vi "AVS_Main.vi"() -> ()   [LabVIEW 2009]
uses:
  <vilib>/express/express arith-compare/Formula/XNode/ExpressFormulaBlockNode.xnode
  Instance           4 16Saved   AVS_Main .vi
  Instance           6 16Saved   AVS_Main .vi
  Instance           5 16Saved   AVS_Main .vi
panel:
  out "a_hDevice":i32
  out "StartTime":u32
  out "XY Graph":cluster{"Y":dbl[], "Y":dbl[]}[](graph)
  out "LastScanTime":dbl caption="Last scan in [ms]" format="%#4.2f"
  out "AvgTimePerScan":dbl caption="Avg Time /Scan [ms]" format="%#4.2f"
  out "Failures":dbl caption="Nr Of Failures" format="%#.0f"
  out "PerformedScans":dbl caption="Nr Of Scans" format="%#.0f"
  out "TotalTime":dbl caption="Time Since Start [s]" format="%#.1f"
  in  "StopMeasurement":bool
  out "Status":string
  in  "StartMeasurement":bool caption="Start Measurement"
  in  "NrOfScans":i16 caption="Nr Of Scans"
  in  "RamSpectra":u16 caption="Spectra stored to RAM"
  in  "LaserWavelenght":sgl caption="Laser Wavelenght [nm]" format="%.2f"
  in  "LaserWidth":u32 caption="Laser Width [ns]"
  in  "LaserDelay":u32 caption="Laser Delay [ns]"
  in  "FlashesPerScan":u16 caption="Flashes per Scan"
  in  "SmoothModel":u8 caption="Model"
  in  "SmoothPix":u16 caption="Nr Of Pixels"
  in  "EnableDarkCorrection":bool caption="Enable"
  in  "DarkHist":u8 caption="%"
  in  "SatDetection":u8 caption="Saturation detection"
  in  "NrOfAVG":u32 caption="Number of averages"
  in  "IntDelay":dbl caption="Integration delay [ns]" min=-20.0 format="%#.0f"
  in  "IntTime":sgl caption="Integration time [ms]" format="%.2f"
  in  "StartPixel":u16 caption="Start pixel"
  in  "StopPixel":u16 caption="Stop pixel"
  in  "Trigger type":enum32{"Radio Selection 1", "Radio Selection 2"}(radio)
  in  "Trigger source":enum32{"Radio Selection 1", "Radio Selection 2"}(radio)
  in  "Trigger mode":T1(radio)
  out "DllVersion":string caption="AvaSpec Dll Version"
  out "FWVersion":string caption="AvaSpec FW Version"
  out "FPGAVersion":string caption="FPGA Version"
  out "NrOfPixel":u16 caption="Nr Of Pixels"
  out "Detector":string
  in  "Exit":bool
  in  "WriteMeasToEEProm":bool
  in  "ReadMeasFromEEProm":bool
  in  "AnalogIO":bool
  in  "DigitalIO":bool
  # "Dark Correction Settings"
  # "Measure"
  # "(-1 = infinite)"
  # "Smoothing Settings"
  # "Control Settings"
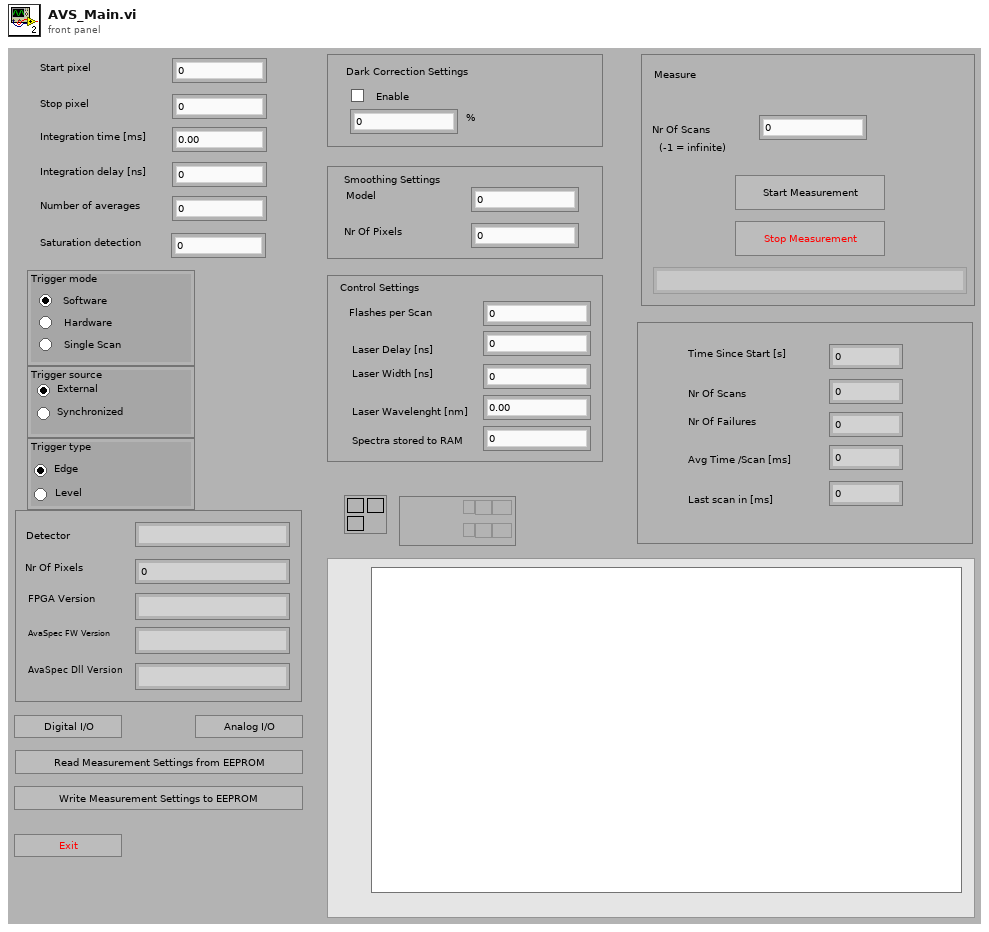
[diagram p1: front panel]
types:
  T1 = enum32{"Radio Selection 2", "Radio Selection 1", "Radio Selection 3"}
  T2 = cluster{"Len":u16, "ConfigVersion":u16, "UserFriendlyId":u8[], "DetectorType":cluster{"SensorType":u8, "NrPixels":u16, "Fit":sgl[], "NLEnable":u8, "NLCorrect":dbl[], "LowNLCounts":dbl, "HighNLCounts":dbl, "Gain":sgl[], "Reserved":sgl, "Offset":sgl[], "Extern Offset":sgl, "DefectivePixels":u16[]}, "IrradianceType":cluster{"SpectrumCalibrationType":cluster{"SmoothingType":cluster{"m_SmoothPix":u16, "SmoothModel":u8}, "CalInttime":sgl, "CalibConvers":sgl[]}, "CalibrationType":u8, "FiberDiameter":i32}, "SpectrumCalibrationType":cluster{"SmoothingType":cluster{"m_SmoothPix":u16, "SmoothModel":u8}, "CalInttime":sgl, "CalibConvers":sgl[]}, "SpectrumCorrectionType":sgl[], "StandAloneType":cluster{"StandAloneType":u8, "MeasConfigType":cluster{"StartPixel":u16, "StopPixel":u16, "IntegrationTime":sgl, "IntegrationDelay":u32, "NrAverages":u32, "DarkCorrectionType":cluster{"Enable CorDynDark":u8, "ForgetPercentage":u8}, "SmoothingType":cluster{"SmoothPix":u16, "SmoothModel":u8}, "SatDetection":u8, "TriggerType":cluster{"Trigger Mode":u8, "Trigger Source":u8, "Trigger SourceType":u8}, "ControlSettingsType":cluster{"StrobeControl":u16, "LaserDelay":u32, "LaserWidth":u32, "LaserWaveLength":sgl, "StoreToRam":u16}}, "Nmsr":i16}, "DynamicStorageType":cluster{"Nmsr":i32, "Reserved":u8[]}, "TempSensorType":sgl[], "TecControlType":cluster{"Enable":u8, "Setpoint":sgl, "Fit[NR_DAC_POL_COEF]":sgl[]}, "ProcessControlType":cluster{"AnalogLow":sgl[], "AnalogHigh":sgl[], "DigitalLow":sgl[], "DigitalHigh":sgl[]}, "EthernetSettingsType":cluster{"IpAddr":u32, "NetMask":u32, "Gateway":u32, "DhcpEnabled":u8, "TcpPort":u16, "LinkStatus":u8}, "Reserved":u8[], "OemData":u8[]}
  T3 = cluster{"StartPixel":u16, "StopPixel":u16, "IntegrationTime":sgl, "IntegrationDelay":u32, "NrAverages":u32, "DarkCorrectionType":cluster{"Enable CorDynDark":u8, "ForgetPercentage":u8}, "SmoothingType":cluster{"SmoothPix":u16, "SmoothModel":u8}, "SatDetection":u8, "TriggerType":cluster{"Trigger Mode":u8, "Trigger Source":u8, "Trigger SourceType":u8}, "ControlSettingsType":cluster{"StrobeControl":u16, "LaserDelay":u32, "LaserWidth":u32, "LaserWaveLength":sgl, "StoreToRam":u16}}
  T4 = cluster{"FlashesPerScan":u16, "Result":u32, "Result":u32, "LaserWavelenght":sgl, "RamSpectra":u16}
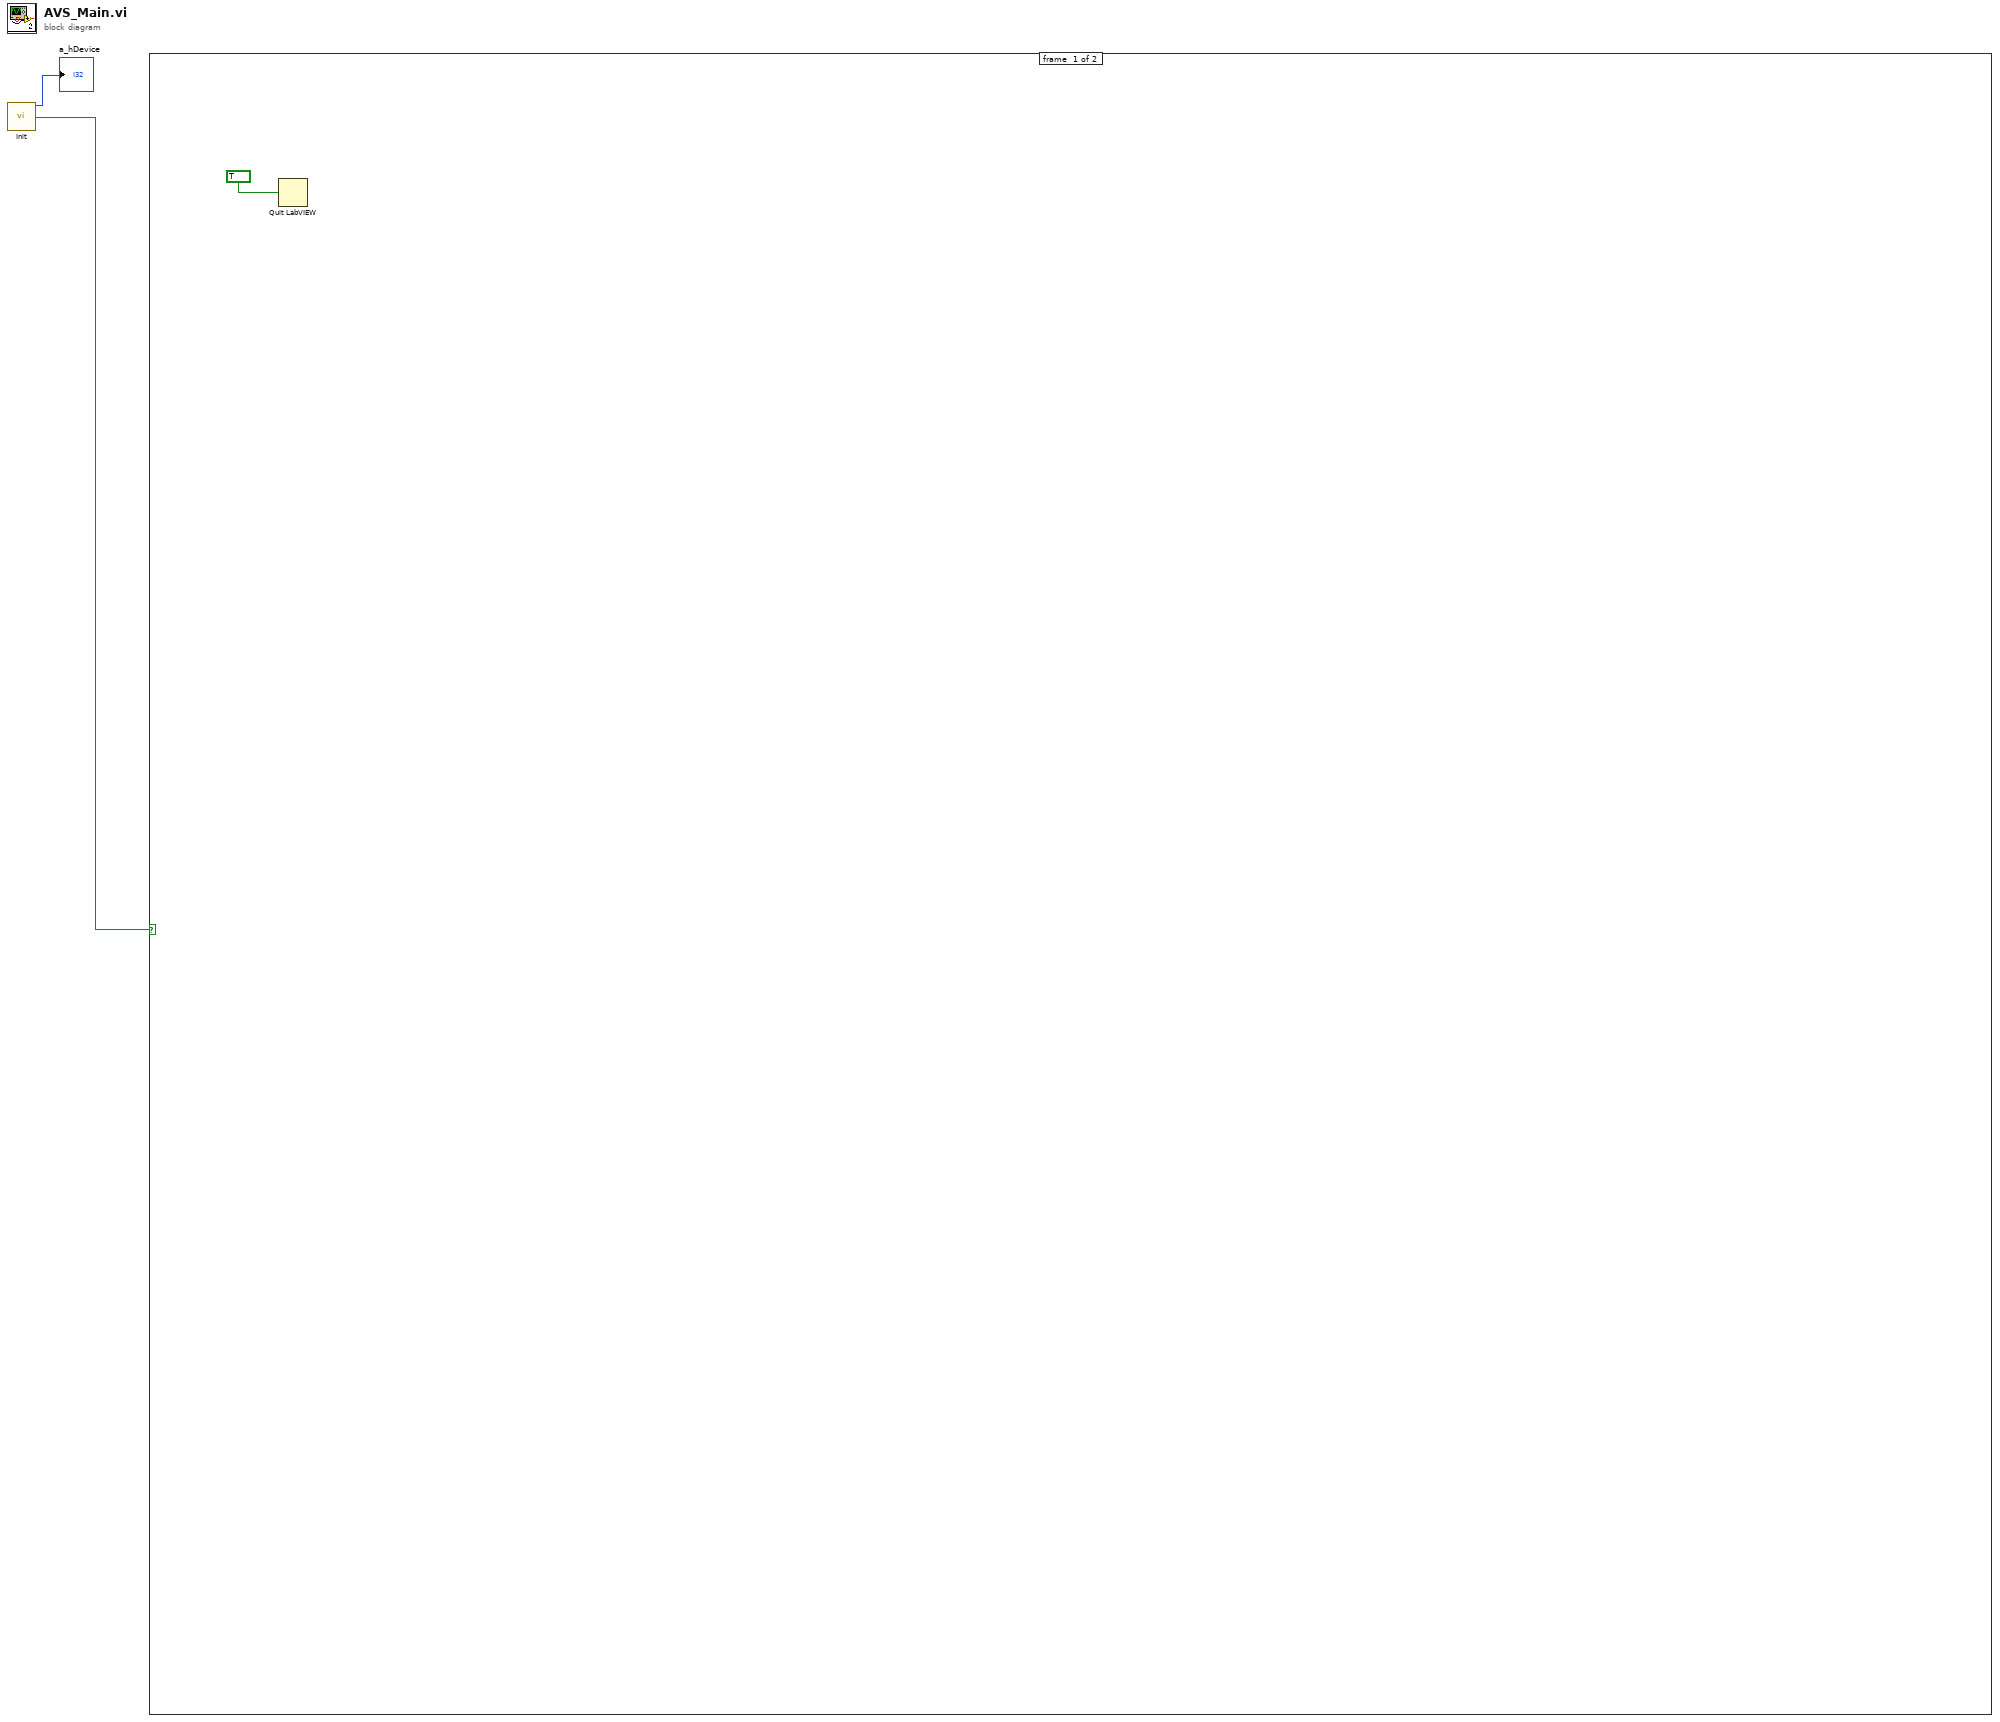
[diagram p0: block diagram]
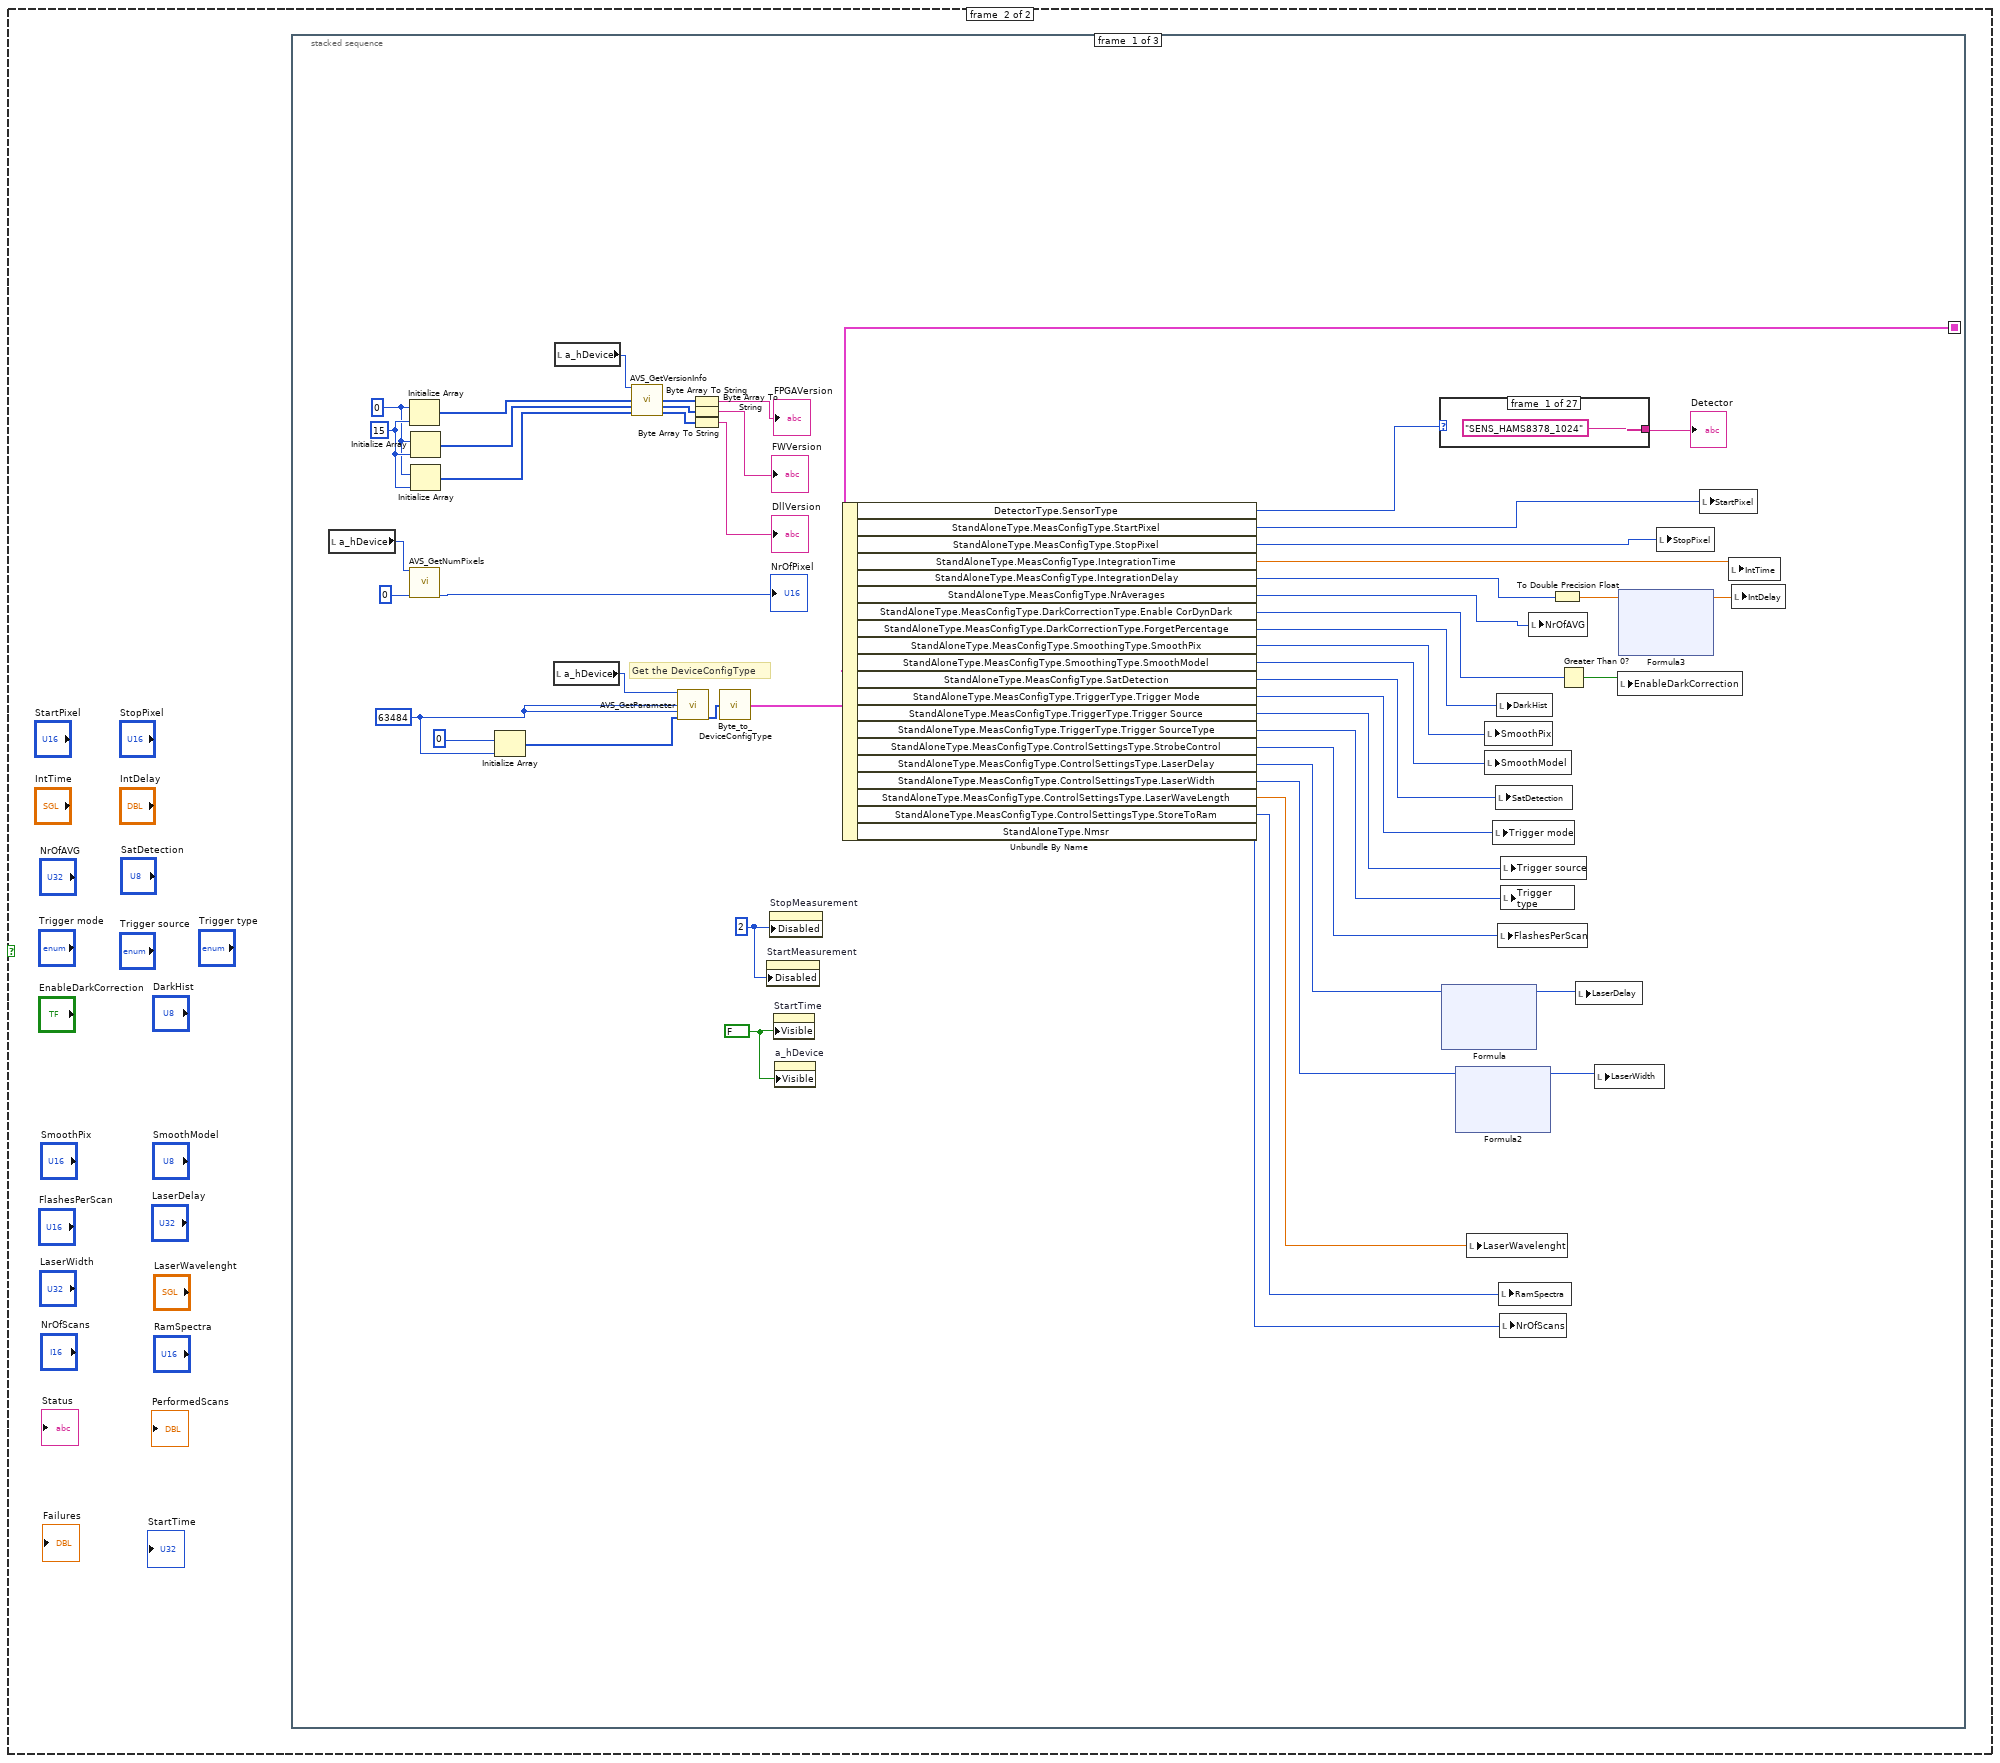
[diagram p2: hidden frame]
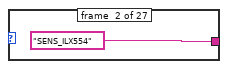
[diagram p3: hidden frame]
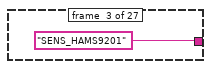
[diagram p4: hidden frame]
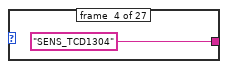
[diagram p5: hidden frame]
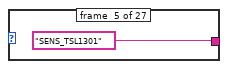
[diagram p6: hidden frame]
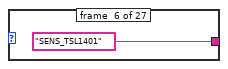
[diagram p7: hidden frame]
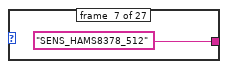
[diagram p8: hidden frame]
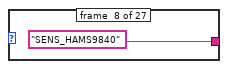
[diagram p9: hidden frame]
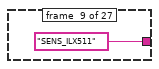
[diagram p10: hidden frame]
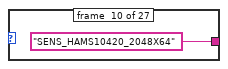
[diagram p11: hidden frame]
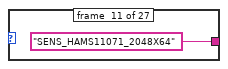
[diagram p12: hidden frame]
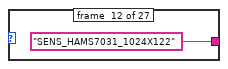
[diagram p13: hidden frame]
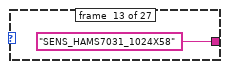
[diagram p14: hidden frame]
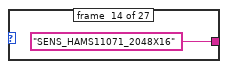
[diagram p15: hidden frame]
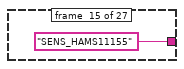
[diagram p16: hidden frame]
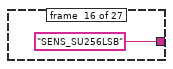
[diagram p17: hidden frame]
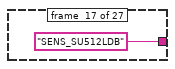
[diagram p18: hidden frame]
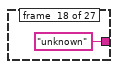
[diagram p19: hidden frame]
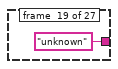
[diagram p20: hidden frame]
diagram:
  n1 = call "Init.vi"() -> ("a_hDevice"=→"a_hDevice":i32, "Aviable"=w2:bool)  [unwired: 14 in]
  n2 = case shown="True" w2 {
    frame #0 {
      n3 = Quit LabVIEW(quit? (T)=TRUE) -> ()
    }
    frame #1 {
      n4 = stacked-sequence {
        seq-local: [w9 _ _] -> [_ w104 _]
        frame #0 {
          w4 = FALSE
          w40 = u8 2 ("Disabled")
          w39 = u16 63484 ("a_pNumPixelsInput")
          w44 = u8 0
          w45 = u16 15 ("a_pNumPixelsInput")
          # "Get the DeviceConfigType"
          n5 = local read "a_hDevice"() -> (w8:i32)
          n6 = Initialize Array(w44, w45) -> (w48:u8[])
          n7 = call "AVS_GetNumPixels.vi"("a_hDevice"=w8, "a_pNumPixels"=u16 0 ("a_pNumPixelsInput")) -> ("a_pNumPixels"=→"NrOfPixel":u16)  [unwired: 12 in, 1 out]
          n8 = Initialize Array(w44, w45) -> (w47:u8[])
          n9 = Initialize Array(w44, w45) -> (w46:u8[])
          n10 = Initialize Array(u8 0, w39) -> (w38:u8[])
          n11 = local read "a_hDevice"() -> (w6:i32)
          n12 = local read "a_hDevice"() -> (w7:i32)
          n13 = call "AVS_GetVersionInfo.vi"("a_hDevice"=w7, "a_pFPGAVersion"=w48, "a_pFirmwareVersion"=w47, "a_pDLLVersion"=w46) -> ("a_pFPGAVersion"=w52:i8[], "a_pFirmwareVersion"=w51:i8[], "a_pDLLVersion"=w50:i8[])  [unwired: 8 in, 1 out]
          n14 = call "AVS_GetParameter.vi"("a_hDevice"=w6, "a_Size"=w39, "RequiredSizeInput"=w39, "DeviceParm"=w38) -> ("DeviceParam"=w37:u8[])  [unwired: 9 in, 2 out]
          n15 = Byte Array To String(unsigned byte array=w52) -> (string=→"FPGAVersion":string)
          n16 = Byte Array To String(unsigned byte array=w51) -> (string=→"FWVersion":string)
          n17 = Byte Array To String(unsigned byte array=w50) -> (string=→"DllVersion":string)
          n18 = call "Byte_to_DeviceConfigType.vi"("Byte Array"=w37) -> ("output cluster"=w9:T2)  [unwired: 4 in]
          n19 = property on="StartMeasurement" class="Bool"("Disabled"=w40) -> ()  [unwired: 2 in, 2 out]
          n20 = property on="StopMeasurement" class="Bool"("Disabled"=w40) -> ()  [unwired: 2 in, 2 out]
          n21 = property on="StartTime" class="DigNum (strict)"("Visible"=w4) -> ()  [unwired: 2 in, 2 out]
          n22 = property on="a_hDevice" class="DigNum (strict)"("Visible"=w4) -> ()  [unwired: 2 in, 2 out]
          n23 = Unbundle By Name(w9) -> ("DetectorType.SensorType"=w34:u8, "StandAloneType.MeasConfigType.StartPixel"=w33:u16, "StandAloneType.MeasConfigType.StopPixel"=w32:u16, "StandAloneType.MeasConfigType.IntegrationTime"=w31:sgl, "StandAloneType.MeasConfigType.IntegrationDelay"=w30:u32, "StandAloneType.MeasConfigType.NrAverages"=w29:u32, "StandAloneType.MeasConfigType.DarkCorrectionType.Enable CorDynDark"=w27:u8, "StandAloneType.MeasConfigType.DarkCorrectionType.ForgetPercentage"=w26:u8, "StandAloneType.MeasConfigType.SmoothingType.SmoothPix"=w25:u16, "StandAloneType.MeasConfigType.SmoothingType.SmoothModel"=w24:u8, "StandAloneType.MeasConfigType.SatDetection"=w23:u8, "StandAloneType.MeasConfigType.TriggerType.Trigger Mode"=w22:u8, "StandAloneType.MeasConfigType.TriggerType.Trigger Source"=w21:u8, "StandAloneType.MeasConfigType.TriggerType.Trigger SourceType"=w20:u8, "StandAloneType.MeasConfigType.ControlSettingsType.StrobeControl"=w19:u16, "StandAloneType.MeasConfigType.ControlSettingsType.LaserDelay"=w18:u32, "StandAloneType.MeasConfigType.ControlSettingsType.LaserWidth"=w17:u32, "StandAloneType.MeasConfigType.ControlSettingsType.LaserWaveLength"=w16:sgl, "StandAloneType.MeasConfigType.ControlSettingsType.StoreToRam"=w15:u16, "StandAloneType.Nmsr"=w14:i16)
          n24 = case shown="26" w34 {
            tunnel: ["SENS_HAMS8378_1024" ("String") "SENS_ILX554" ("String") "SENS_HAMS9201" ("String") "SENS_TCD1304" ("String") "SENS_TSL1301" ("String") "SENS_TSL1401" ("String") "SENS_HAMS8378_512" ("String") "SENS_HAMS9840" ("String") "SENS_ILX511" ("String") "SENS_HAMS10420_2048X64" ("String") "SENS_HAMS11071_2048X64" ("String") "SENS_HAMS7031_1024X122" ("String") "SENS_HAMS7031_1024X58" ("String") "SENS_HAMS11071_2048X16" ("String") "SENS_HAMS11155" ("String") "SENS_SU256LSB" ("String") "SENS_SU512LDB" ("String") "unknown" ("String") "unknown" ("String") "SENS_HAMS11638" ("String") "SENS_HAMS11639" ("String") "SENS_HAMS12443" ("String") "SENS_HAMG9208_512" ("String") "SENS_HAMG13913" ("String") "SENS_HAMS13496" ("String") "unknown" ("String") "SENS_HAMS8378_256" ("String")] -> w5
            frame #0 {
            }
            frame #1 {
            }
            frame #2 {
            }
            frame #3 {
            }
            frame #4 {
            }
            frame #5 {
            }
            frame #6 {
            }
            frame #7 {
            }
            frame #8 {
            }
            frame #9 {
            }
            frame #10 {
            }
            frame #11 {
            }
            frame #12 {
            }
            frame #13 {
            }
            frame #14 {
            }
            frame #15 {
            }
            frame #16 {
            }
            frame #17 {
            }
            frame #18 {
            }
            frame #19 {
            }
            frame #20 {
            }
            frame #21 {
            }
            frame #22 {
            }
            frame #23 {
            }
            frame #24 {
            }
            frame #25 {
            }
            frame #26 {
            }
          }
          "Detector" <- w5
          n25 = xnode "Formula"("X1"=w18) -> ("Result"=w42:u32)  [unwired: 1 in, 1 out]
          n26 = xnode "Formula2"("X1"=w17) -> ("Result"=w41:u32)  [unwired: 1 in, 1 out]
          n27 = local write "LaserWavelenght"(w16) -> ()
          n28 = local write "SmoothPix"(w25) -> ()
          n29 = local write "SmoothModel"(w24) -> ()
          n30 = local write "Trigger mode"(w22) -> ()
          n31 = local write "SatDetection"(w23) -> ()
          n32 = local write "DarkHist"(w26) -> ()
          n33 = local write "FlashesPerScan"(w19) -> ()
          n34 = local write "RamSpectra"(w15) -> ()
          n35 = local write "NrOfScans"(w14) -> ()
          n36 = local write "Trigger source"(w21) -> ()
          n37 = local write "Trigger type"(w20) -> ()
          n38 = local write "NrOfAVG"(w29) -> ()
          n39 = To Double Precision Float(number=w30) -> (double precision float=w36:dbl)
          n40 = Greater Than 0?(x=w27) -> (x > 0?=w28:bool)
          n41 = local write "LaserDelay"(w42) -> ()
          n42 = local write "LaserWidth"(w41) -> ()
          n43 = local write "EnableDarkCorrection"(w28) -> ()
          n44 = xnode "Formula3"("X1"=w36) -> ("Result"=w35:dbl)  [unwired: 1 in, 1 out]
          n45 = local write "StopPixel"(w32) -> ()
          n46 = local write "StartPixel"(w33) -> ()
          n47 = local write "IntTime"(w31) -> ()
          n48 = local write "IntDelay"(w35) -> ()
        }
        frame #1 {
          w105 = u8 0 ("Disabled")
          n49 = property on="StopMeasurement" class="Bool"("Disabled"=w105) -> ()  [unwired: 2 in, 2 out]
          n50 = property on="StartMeasurement" class="Bool"("Disabled"=w105) -> ()  [unwired: 2 in, 2 out]
          n51 = while {
            tunnel: w104 -> [w109]
            shift-right: [w108] -> _
            shift-left: _ -> [w107]
            stop <- w113 stop-if-true
            # "Wait until measurement has finished and new data are available."
            n52 = local read "a_hDevice"() -> (w111:i32)
            n53 = event shown="[5] \"WriteMeasToEEProm\": Value Change" {
              selector: _ -> [_ _ _ _ _ _ _ _]
              dyn-events: _ -> [_ _ _ _ _ _ _ _]
              timeout: 1 -> [_ _ _ _ _ _ _ _]
              tunnel: [_ _ _ _ _ _ _ "Exit"] -> w113
              tunnel: w109 -> [_ _ _ _ _ w324 _ _]
              event #0 {
                n54 = event-data() -> ()  [unwired: 1 in, 2 out]
              }
              event #1 {
                w192 = T3 {"StartPixel"=0, "StopPixel"=0, "IntegrationTime"=0.0, "IntegrationDelay"=0, "NrAverages"=0, "DarkCorrectionType"={"Enable CorDynDark"=0, "ForgetPercentage"=0}, "SmoothingType"={"SmoothPix"=0, "SmoothModel"=0}, "SatDetection"=0, "TriggerType"={"Trigger Mode"=0, "Trigger Source"=0, "Trigger SourceType"=0}, "ControlSettingsType"={"StrobeControl"=0, "LaserDelay"=0, "LaserWidth"=0, "LaserWaveLength"=0.0, "StoreToRam"=0}}  # MeasConfigType
                w174 = u8 2 ("Disabled")
                w198 = 0.0 ("Failures")
                # "StartMeas:\n1: Prepares measurement on the spectrometer \nusing the specified measurement configuration. \n2: Start measurement"
                n55 = event-data() -> ()  [unwired: 1 in, 6 out]
                n56 = local read "EnableDarkCorrection"() -> (w199:bool)
                n57 = local read "SmoothModel"() -> (w187:u8)
                n58 = local read "Trigger mode"() -> (w201:T1)
                n59 = local read "Trigger source"() -> (w202:enum32{"Radio Selection 1", "Radio Selection 2"})
                n60 = local read "SmoothPix"() -> (w188:u16)
                n61 = local read "SatDetection"() -> (w184:u8)
                n62 = local read "Trigger type"() -> (w200:enum32{"Radio Selection 1", "Radio Selection 2"})
                n63 = local read "FlashesPerScan"() -> (w175:u16)
                n64 = local read "LaserWavelenght"() -> (w178:sgl)
                n65 = local read "RamSpectra"() -> (w179:u16)
                n66 = local read "LaserWidth"() -> (w193:u32)
                n67 = local read "DarkHist"() -> (w190:u8)
                n68 = local read "LaserDelay"() -> (w194:u32)
                n69 = local read "IntTime"() -> (w204:sgl)
                n70 = local read "StartPixel"() -> (w206:u16)
                n71 = local read "StopPixel"() -> (w205:u16)
                n72 = local read "NrOfAVG"() -> (w207:u32)
                n73 = local read "IntDelay"() -> (w195:dbl)
                n74 = xnode "Formula6"("X1"=w193) -> ("Result"=w177:u32)  [unwired: 1 in, 1 out]
                n75 = xnode "Formula5"("X1"=w194) -> ("Result"=w176:u32)  [unwired: 1 in, 1 out]
                n76 = Boolean To (0,1)(Boolean=w199) -> (0, 1=w203:i16)
                n77 = Bundle("SmoothPix"=w188, "SmoothModel"=w187) -> (w186:cluster{"SmoothPix":u16, "SmoothModel":u8})  [unwired: 1 in]
                n78 = xnode "Formula4"("X1"=w195) -> ("Result"=w196:dbl)  [unwired: 1 in, 1 out]
                n79 = To Unsigned Byte Integer(number=w203) -> (unsigned 8bit integer=w191:u8)
                n80 = To Unsigned Byte Integer(number=w202) -> (unsigned 8bit integer=w182:u8)
                n81 = Bundle(w191, "DarkHist"=w190) -> (w189:cluster{u8, "DarkHist":u8})  [unwired: 1 in]
                n82 = To Unsigned Byte Integer(number=w201) -> (unsigned 8bit integer=w185:u8)
                n83 = To Unsigned Byte Integer(number=w200) -> (unsigned 8bit integer=w183:u8)
                n84 = To Unsigned Long Integer(number=w196) -> (unsigned 32bit integer=w197:u32)
                n85 = Bundle("FlashesPerScan"=w175, "Result"=w176, "Result"=w177, "LaserWavelenght"=w178, "RamSpectra"=w179) -> (w180:T4)  [unwired: 1 in]
                n86 = Bundle(w185, w182, w183) -> (w181:cluster{u8, u8, u8})  [unwired: 1 in]
                n87 = Bundle(cluster=w192, "StartPixel"=w206, "StopPixel"=w205, "IntegrationTime"=w204, "IntegrationDelay"=w197, "NrAverages"=w207, "DarkCorrectionType"=w189, "SmoothingType"=w186, "SatDetection"=w184, "TriggerType"=w181, "ControlSettingsType"=w180) -> (w208:T3)
                n88 = local write "Failures"(w198) -> ()
                n89 = local write "TotalTime"(w198) -> ()
                n90 = local write "PerformedScans"(w198) -> ()
                n91 = local write "AvgTimePerScan"(w198) -> ()
                n92 = local write "LastScanTime"(w198) -> ()
                n93 = local read "NrOfScans"() -> (w170:i16)
                n94 = local read "a_hDevice"() -> (w171:i32)
                n95 = call "StartMeasurement.vi"("a_hDevice"=w171, "a_hWnd"=0, "a_Nmsr"=w170, "MeasConfigType"=w208) -> ("Status"=w173:string, "StartTime"=w172:u32)  [unwired: 10 in]
                n96 = local write "StartTime"(w172) -> ()
                n97 = property on="StartMeasurement" class="Bool"("Disabled"=w174) -> ()  [unwired: 2 in, 2 out]
                n98 = property on="AnalogIO" class="Bool"("Disabled"=w174) -> ()  [unwired: 2 in, 2 out]
                n99 = property on="DigitalIO" class="Bool"("Disabled"=w174) -> ()  [unwired: 2 in, 2 out]
                n100 = property on="ReadMeasFromEEProm" class="Bool"("Disabled"=w174) -> ()  [unwired: 2 in, 2 out]
                n101 = local write "Status"(w173) -> ()
                n102 = property on="WriteMeasToEEProm" class="Bool"("Disabled"=w174) -> ()  [unwired: 2 in, 2 out]
              }
              event #2 {
                n103 = event-data() -> ()  [unwired: 1 in, 6 out]
                n104 = flat-sequence {
                  frame #0 {
                    w233 = u8 2 ("Disabled")
                    n105 = property on="StopMeasurement" class="Bool"("Disabled"=w233) -> ()  [unwired: 2 in, 2 out]
                    n106 = property on="StartMeasurement" class="Bool"("Disabled"=w233) -> ()  [unwired: 2 in, 2 out]
                    n107 = property on="DigitalIO" class="Bool"("Disabled"=w233) -> ()  [unwired: 2 in, 2 out]
                    n108 = property on="ReadMeasFromEEProm" class="Bool"("Disabled"=w233) -> ()  [unwired: 2 in, 2 out]
                    n109 = property on="WriteMeasToEEProm" class="Bool"("Disabled"=w233) -> ()  [unwired: 2 in, 2 out]
                  }
                  frame #1 {
                    n110 = local read "a_hDevice"() -> (w234:i32)
                    n111 = call "AnalogIO.vi"("a_hDevice"=w234) -> ()  [unwired: 15 in]
                  }
                  frame #2 {
                    w235 = u8 0 ("Disabled")
                    n112 = property on="StopMeasurement" class="Bool"("Disabled"=w235) -> ()  [unwired: 2 in, 2 out]
                    n113 = property on="StartMeasurement" class="Bool"("Disabled"=w235) -> ()  [unwired: 2 in, 2 out]
                    n114 = property on="DigitalIO" class="Bool"("Disabled"=w235) -> ()  [unwired: 2 in, 2 out]
                    n115 = property on="ReadMeasFromEEProm" class="Bool"("Disabled"=w235) -> ()  [unwired: 2 in, 2 out]
                    n116 = property on="WriteMeasToEEProm" class="Bool"("Disabled"=w235) -> ()  [unwired: 2 in, 2 out]
                  }
                }
              }
              event #3 {
                n117 = event-data() -> ()  [unwired: 1 in, 6 out]
                n118 = flat-sequence {
                  frame #0 {
                    w236 = u8 2 ("Disabled")
                    n119 = property on="StartMeasurement" class="Bool"("Disabled"=w236) -> ()  [unwired: 2 in, 2 out]
                    n120 = property on="StopMeasurement" class="Bool"("Disabled"=w236) -> ()  [unwired: 2 in, 2 out]
                    n121 = property on="AnalogIO" class="Bool"("Disabled"=w236) -> ()  [unwired: 2 in, 2 out]
                    n122 = property on="WriteMeasToEEProm" class="Bool"("Disabled"=w236) -> ()  [unwired: 2 in, 2 out]
                    n123 = property on="ReadMeasFromEEProm" class="Bool"("Disabled"=w236) -> ()  [unwired: 2 in, 2 out]
                  }
                  frame #1 {
                    n124 = local read "a_hDevice"() -> (w237:i32)
                    n125 = call "DigitalIO.vi"("a_hDevice"=w237) -> ()  [unwired: 15 in]
                  }
                  frame #2 {
                    w238 = u8 0 ("Disabled")
                    n126 = property on="StopMeasurement" class="Bool"("Disabled"=w238) -> ()  [unwired: 2 in, 2 out]
                    n127 = property on="StartMeasurement" class="Bool"("Disabled"=w238) -> ()  [unwired: 2 in, 2 out]
                    n128 = property on="AnalogIO" class="Bool"("Disabled"=w238) -> ()  [unwired: 2 in, 2 out]
                    n129 = property on="ReadMeasFromEEProm" class="Bool"("Disabled"=w238) -> ()  [unwired: 2 in, 2 out]
                    n130 = property on="WriteMeasToEEProm" class="Bool"("Disabled"=w238) -> ()  [unwired: 2 in, 2 out]
                  }
                }
              }
              event #4 {
                n131 = event-data() -> ()  [unwired: 1 in, 6 out]
                n132 = stacked-sequence {
                  frame #0 {
                    w239 = u8 2 ("Disabled")
                    n133 = property on="StartMeasurement" class="Bool"("Disabled"=w239) -> ()  [unwired: 2 in, 2 out]
                    n134 = property on="StopMeasurement" class="Bool"("Disabled"=w239) -> ()  [unwired: 2 in, 2 out]
                    n135 = property on="AnalogIO" class="Bool"("Disabled"=w239) -> ()  [unwired: 2 in, 2 out]
                    n136 = property on="WriteMeasToEEProm" class="Bool"("Disabled"=w239) -> ()  [unwired: 2 in, 2 out]
                    n137 = property on="DigitalIO" class="Bool"("Disabled"=w239) -> ()  [unwired: 2 in, 2 out]
                  }
                  frame #1 {
                    w271 = u16 63484 ("a_pNumPixelsInput")
                    n138 = local read "a_hDevice"() -> (w240:i32)
                    n139 = Initialize Array(u8 0, w271) -> (w270:u8[])
                    n140 = call "AVS_GetParameter.vi"("a_hDevice"=w240, "a_Size"=w271, "RequiredSizeInput"=w271, "DeviceParm"=w270) -> ("DeviceParam"=w262:u8[])  [unwired: 9 in, 2 out]
                    n141 = call "Byte_to_DeviceConfigType.vi"("Byte Array"=w262) -> ("output cluster"=w241:T2)  [unwired: 4 in]
                    n142 = Unbundle By Name(w241) -> ("DetectorType.SensorType"=w261:u8, "StandAloneType.MeasConfigType.StartPixel"=w260:u16, "StandAloneType.MeasConfigType.StopPixel"=w259:u16, "StandAloneType.MeasConfigType.IntegrationTime"=w258:sgl, "StandAloneType.MeasConfigType.IntegrationDelay"=w257:u32, "StandAloneType.MeasConfigType.NrAverages"=w256:u32, "StandAloneType.MeasConfigType.DarkCorrectionType.Enable CorDynDark"=w254:u8, "StandAloneType.MeasConfigType.DarkCorrectionType.ForgetPercentage"=w253:u8, "StandAloneType.Nmsr"=w255:i16, "StandAloneType.MeasConfigType.SmoothingType.SmoothPix"=w252:u16, "StandAloneType.MeasConfigType.SmoothingType.SmoothModel"=w251:u8, "StandAloneType.MeasConfigType.SatDetection"=w250:u8, "StandAloneType.MeasConfigType.TriggerType.Trigger Mode"=w249:u8, "StandAloneType.MeasConfigType.TriggerType.Trigger Source"=w248:u8, "StandAloneType.MeasConfigType.TriggerType.Trigger SourceType"=w247:u8, "StandAloneType.MeasConfigType.ControlSettingsType.StrobeControl"=w242:u16, "StandAloneType.MeasConfigType.ControlSettingsType.LaserDelay"=w243:u32, "StandAloneType.MeasConfigType.ControlSettingsType.LaserWidth"=w244:u32, "StandAloneType.MeasConfigType.ControlSettingsType.LaserWaveLength"=w245:sgl, "StandAloneType.MeasConfigType.ControlSettingsType.StoreToRam"=w246:u16)
                    n143 = case shown="26" w261 {
                      tunnel: ["SENS_HAMS8378_1024" ("String") "SENS_ILX554" ("String") "SENS_HAMS9201" ("String") "SENS_TCD1304" ("String") "SENS_TSL1301" ("String") "SENS_TSL1401" ("String") "SENS_HAMS8378_512" ("String") "SENS_HAMS9840" ("String") "SENS_ILX511" "SENS_HAMS10420_2048X64" ("String") "SENS_HAMS11071_2048X64" ("String") "SENS_HAMS7031_1024X122" ("String") "SENS_HAMS7031_1024X58" ("String") "SENS_HAMS11071_2048X16" ("String") "SENS_HAMS11155" ("String") "SENS_SU256LSB" ("String") "SENS_SU512LDB" ("String") "unknown" ("String") "unknown" ("String") "SENS_HAMS11638" ("String") "SENS_HAMS11639" ("String") "SENS_HAMS12443" ("String") "SENS_HAMG9208_512" ("String") "SENS_HAMG13913" ("String") "SENS_HAMS13496" ("String") "unknown" ("String") "SENS_HAMS8378_256" ("String")] -> w268
                      frame #0 {
                      }
                      frame #1 {
                      }
                      frame #2 {
                      }
                      frame #3 {
                      }
                      frame #4 {
                      }
                      frame #5 {
                      }
                      frame #6 {
                      }
                      frame #7 {
                      }
                      frame #8 {
                      }
                      frame #9 {
                      }
                      frame #10 {
                      }
                      frame #11 {
                      }
                      frame #12 {
                      }
                      frame #13 {
                      }
                      frame #14 {
                      }
                      frame #15 {
                      }
                      frame #16 {
                      }
                      frame #17 {
                      }
                      frame #18 {
                      }
                      frame #19 {
                      }
                      frame #20 {
                      }
                      frame #21 {
                      }
                      frame #22 {
                      }
                      frame #23 {
                      }
                      frame #24 {
                      }
                      frame #25 {
                      }
                      frame #26 {
                      }
                    }
                    n144 = To Double Precision Float(number=w257) -> (double precision float=w263:dbl)
                    n145 = local write "Trigger mode"(w249) -> ()
                    n146 = local write "IntTime"(w258) -> ()
                    n147 = local write "NrOfAVG"(w256) -> ()
                    n148 = xnode "Formula7"("X1"=w243) -> ("Result"=w265:u32)  [unwired: 1 in, 1 out]
                    n149 = xnode "Formula8"("X1"=w244) -> ("Result"=w264:u32)  [unwired: 1 in, 1 out]
                    n150 = local write "Trigger type"(w247) -> ()
                    n151 = local write "FlashesPerScan"(w242) -> ()
                    n152 = local write "RamSpectra"(w246) -> ()
                    n153 = local write "LaserWavelenght"(w245) -> ()
                    n154 = local write "SmoothPix"(w252) -> ()
                    n155 = local write "NrOfScans"(w255) -> ()
                    n156 = local write "SatDetection"(w250) -> ()
                    n157 = Greater Than 0?(x=w254) -> (x > 0?=w267:bool)
                    n158 = xnode "Formula9"("X1"=w263) -> ("Result"=w266:dbl)  [unwired: 1 in, 1 out]
                    n159 = local write "EnableDarkCorrection"(w267) -> ()
                    n160 = local write "StopPixel"(w259) -> ()
                    n161 = local write "StartPixel"(w260) -> ()
                    n162 = local write "SmoothModel"(w251) -> ()
                    n163 = local write "Trigger source"(w248) -> ()
                    n164 = local write "DarkHist"(w253) -> ()
                    n165 = local write "LaserDelay"(w265) -> ()
                    n166 = local write "LaserWidth"(w264) -> ()
                    n167 = local write "IntDelay"(w266) -> ()
                    n168 = local write "Detector"(w268) -> ()
                  }
                  frame #2 {
                    w323 = u8 0 ("Disabled")
                    n169 = property on="StopMeasurement" class="Bool"("Disabled"=w323) -> ()  [unwired: 2 in, 2 out]
                    n170 = property on="AnalogIO" class="Bool"("Disabled"=w323) -> ()  [unwired: 2 in, 2 out]
                    n171 = property on="DigitalIO" class="Bool"("Disabled"=w323) -> ()  [unwired: 2 in, 2 out]
                    n172 = property on="StartMeasurement" class="Bool"("Disabled"=w323) -> ()  [unwired: 2 in, 2 out]
                    n173 = property on="WriteMeasToEEProm" class="Bool"("Disabled"=w323) -> ()  [unwired: 2 in, 2 out]
                  }
                }
              }
              event #5 {
                n174 = event-data() -> ()  [unwired: 1 in, 6 out]
                n175 = stacked-sequence {
                  tunnel: w324 -> [_ w327 _]
                  frame #0 {
                    w325 = u8 2 ("Disabled")
                    n176 = property on="StopMeasurement" class="Bool"("Disabled"=w325) -> ()  [unwired: 2 in, 2 out]
                    n177 = property on="ReadMeasFromEEProm" class="Bool"("Disabled"=w325) -> ()  [unwired: 2 in, 2 out]
                    n178 = property on="AnalogIO" class="Bool"("Disabled"=w325) -> ()  [unwired: 2 in, 2 out]
                    n179 = property on="DigitalIO" class="Bool"("Disabled"=w325) -> ()  [unwired: 2 in, 2 out]
                    n180 = property on="StartMeasurement" class="Bool"("Disabled"=w325) -> ()  [unwired: 2 in, 2 out]
                  }
                  frame #1 {
                    n181 = local read "NrOfAVG"() -> (w338:u32)
                    n182 = local read "DarkHist"() -> (w340:u8)
                    n183 = local read "StartPixel"() -> (w334:u16)
                    n184 = local read "StopPixel"() -> (w335:u16)
                    n185 = local read "IntTime"() -> (w336:sgl)
                    n186 = local read "IntDelay"() -> (w337:dbl)
                    n187 = local read "SmoothModel"() -> (w342:u8)
                    n188 = local read "NrOfScans"() -> (w354:i16)
                    n189 = local read "SmoothPix"() -> (w341:u16)
                    n190 = local read "Trigger mode"() -> (w344:T1)
                    n191 = local read "Trigger type"() -> (w346:enum32{"Radio Selection 1", "Radio Selection 2"})
                    n192 = local read "LaserDelay"() -> (w348:u32)
                    n193 = local read "LaserWidth"() -> (w349:u32)
                    n194 = local read "SatDetection"() -> (w343:u8)
                    n195 = local read "Trigger source"() -> (w345:enum32{"Radio Selection 1", "Radio Selection 2"})
                    n196 = local read "FlashesPerScan"() -> (w347:u16)
                    n197 = local read "RamSpectra"() -> (w353:u16)
                    n198 = local read "LaserWavelenght"() -> (w352:sgl)
                    n199 = local read "EnableDarkCorrection"() -> (w339:bool)
                    n200 = local read "Detector"() -> (w333:string)
                    n201 = xnode "Formula11"("X1"=w349) -> ("Result"=w351:u32)  [unwired: 1 in, 1 out]
                    n202 = case shown="\"SENS_HAMS13496\"" w333 {
                      tunnel: [2 3 4 5 6 7 8 9 10 11 12 13 14 15 16 17 18 21 22 23 24 25 26 0 1] -> w329
                      frame #0 {
                      }
                      frame #1 {
                      }
                      frame #2 {
                      }
                      frame #3 {
                      }
                      frame #4 {
                      }
                      frame #5 {
                      }
                      frame #6 {
                      }
                      frame #7 {
                      }
                      frame #8 {
                      }
                      frame #9 {
                      }
                      frame #10 {
                      }
                      frame #11 {
                      }
                      frame #12 {
                      }
                      frame #13 {
                      }
                      frame #14 {
                      }
                      frame #15 {
                      }
                      frame #16 {
                      }
                      frame #17 {
                      }
                      frame #18 {
                      }
                      frame #19 {
                      }
                      frame #20 {
                      }
                      frame #21 {
                      }
                      frame #22 {
                      }
                      frame #23 {
                      }
                      frame #24 {
                      }
                    }
                    n203 = xnode "Formula12"("X1"=w337) -> ("Result"=w332:dbl)  [unwired: 1 in, 1 out]
                    n204 = xnode "Formula10"("X1"=w348) -> ("Result"=w350:u32)  [unwired: 1 in, 1 out]
                    n205 = Boolean To (0,1)(Boolean=w339) -> ()  [unwired: 1 out]
                    n206 = To Unsigned Long Integer(number=w332) -> (unsigned 32bit integer=w331:u32)
                    n207 = Bundle By Name(cluster=w327, "DetectorType.SensorType"=w329) -> (w330:T2)
                    n208 = Bundle By Name(cluster=w330, "StandAloneType.MeasConfigType.StartPixel"=w334, "StandAloneType.MeasConfigType.StopPixel"=w335, "StandAloneType.MeasConfigType.IntegrationTime"=w336, "StandAloneType.MeasConfigType.IntegrationDelay"=w331, "StandAloneType.MeasConfigType.NrAverages"=w338, "StandAloneType.MeasConfigType.DarkCorrectionType.ForgetPercentage"=w340, "StandAloneType.MeasConfigType.SmoothingType.SmoothPix"=w341, "StandAloneType.MeasConfigType.SmoothingType.SmoothModel"=w342, "StandAloneType.MeasConfigType.SatDetection"=w343, "StandAloneType.MeasConfigType.TriggerType.Trigger Mode"=w344, "StandAloneType.MeasConfigType.TriggerType.Trigger Source"=w345, "StandAloneType.MeasConfigType.TriggerType.Trigger SourceType"=w346, "StandAloneType.MeasConfigType.ControlSettingsType.StrobeControl"=w347, "StandAloneType.MeasConfigType.ControlSettingsType.LaserDelay"=w350, "StandAloneType.MeasConfigType.ControlSettingsType.LaserWidth"=w351, "StandAloneType.MeasConfigType.ControlSettingsType.LaserWaveLength"=w352, "StandAloneType.MeasConfigType.ControlSettingsType.StoreToRam"=w353, "StandAloneType.Nmsr"=w354) -> (w326:T2)
                    n209 = call "DeviceConfigType_to_Byte.vi"("DeviceConfig"=w326) -> ("Byte Array"=w355:u8[])  [unwired: 4 in]
                    n210 = local read "a_hDevice"() -> (w328:i32)
                    n211 = call "AVS_SetParameter.vi"("a_hDevice"=w328, "a_pDeviceParm"=w355) -> ()  [unwired: 12 in, 2 out]
                  }
                  frame #2 {
                    w405 = u8 0 ("Disabled")
                    n212 = property on="StopMeasurement" class="Bool"("Disabled"=w405) -> ()  [unwired: 2 in, 2 out]
                    n213 = property on="ReadMeasFromEEProm" class="Bool"("Disabled"=w405) -> ()  [unwired: 2 in, 2 out]
                    n214 = property on="StartMeasurement" class="Bool"("Disabled"=w405) -> ()  [unwired: 2 in, 2 out]
                    n215 = property on="DigitalIO" class="Bool"("Disabled"=w405) -> ()  [unwired: 2 in, 2 out]
                    n216 = property on="AnalogIO" class="Bool"("Disabled"=w405) -> ()  [unwired: 2 in, 2 out]
                  }
                }
              }
              event #6 {
                w407 = u8 0 ("Disabled")
                n217 = event-data() -> ()  [unwired: 1 in, 6 out]
                n218 = local read "a_hDevice"() -> (w406:i32)
                n219 = property on="StartMeasurement" class="Bool"("Disabled"=w407) -> ()  [unwired: 2 in, 2 out]
                n220 = property on="AnalogIO" class="Bool"("Disabled"=w407) -> ()  [unwired: 2 in, 2 out]
                n221 = property on="DigitalIO" class="Bool"("Disabled"=w407) -> ()  [unwired: 2 in, 2 out]
                n222 = property on="ReadMeasFromEEProm" class="Bool"("Disabled"=w407) -> ()  [unwired: 2 in, 2 out]
                n223 = property on="WriteMeasToEEProm" class="Bool"("Disabled"=w407) -> ()  [unwired: 2 in, 2 out]
                n224 = call "AVS_StopMeasure.vi"("a_hDevice"=w406) -> ()  [unwired: 14 in, 1 out]
              }
              event #7 {
                n225 = event-data() -> ()  [unwired: 1 in, 6 out]
              }
            }
            n226 = call "AVS_PollScan.vi"("a_hDevice"=w111) -> ("Output Value"=w110:i32)  [unwired: 8 in]
            n227 = Less Than 0?(x=w110) -> (x < 0?=w112:bool)
            n228 = case shown="True" w112 {
              tunnel: w110 -> [_ w166]
              frame #0 {
              }
              frame #1 {
                n229 = Number To Decimal String(number=w166) -> (decimal integer string=w165:string)  [unwired: 1 in]
                n230 = Concatenate Strings("Error code: ", w165) -> (w168:string)
                n231 = local write "Status"(w168) -> ()
              }
            }
            n232 = case shown="1" w110 {
              tunnel: [w114 w116] -> w108
              tunnel: w107 -> [w114 w115]
              frame #0 {
              }
              frame #1 {
                n233 = stacked-sequence {
                  seq-local: [_ w143 _] -> [_ _ w151]
                  tunnel: [_ w137 _] -> w120
                  tunnel: [w126 _ _] -> w117
                  tunnel: [_ w139 _] -> w116
                  tunnel: w115 -> [_ w138 _]
                  frame #0 {
                    n234 = local read "StopPixel"() -> (w124:u16)
                    n235 = local read "StartPixel"() -> (w123:u16)
                    n236 = local read "a_hDevice"() -> (w130:i32)
                    n237 = Subtract(x=w124, y=w123) -> (x-y=w122:u16)
                    n238 = Initialize Array(0.0, 4096 ("dimension size")) -> (w128:dbl[])
                    n239 = local read "StartPixel"() -> (w125:u16)
                    n240 = call "AVS_GetLambda.vi"("a_hDevice"=w130, "a_pWaveLength"=w128) -> ("a_pWaveLength"=w127:dbl[])  [unwired: 12 in, 1 out]
                    n241 = Array Subset(array=w127, index=w125, length=w122) -> (w126:dbl[])
                  }
                  frame #1 {
                    # "Returns the values for each pixel"
                    n242 = local read "StopPixel"() -> (w134:u16)
                    n243 = local read "StartPixel"() -> (w133:u16)
                    n244 = local read "a_hDevice"() -> (w142:i32)
                    n245 = local read "PerformedScans"() -> (w149:dbl)
                    n246 = Subtract(x=w134, y=w133) -> (x-y=w132:u16)
                    n247 = Initialize Array(0.0 ("element"), 4096 ("dimension size")) -> (w147:dbl[])
                    n248 = call "AVS_GetScopeData.vi"("a_hDevice"=w142, "a_pTimeLabel"=u32 0, "a_pSpectrum"=w147) -> ("a_pTimeLabel"=w139:u32, "a_pSpectrum"=w136:dbl[])  [unwired: 10 in, 1 out]
                    n249 = Array Subset(array=w136, index=0, length=w132) -> (w137:dbl[])
                    n250 = Increment(x=w149) -> (x+1=w150:dbl)
                    n251 = local write "Status"("Meas.Status: success" ("Status")) -> ()
                    n252 = local write "PerformedScans"(w150) -> ()
                    n253 = Subtract(x=w139, y=w138) -> (x-y=w140:u32)
                    n254 = Divide(x=w140, y=u32 100) -> (x/y=w143:dbl)
                  }
                  frame #2 {
                    n255 = Tick Count (ms)() -> (millisecond timer value=w163:u32)
                    n256 = local read "StartTime"() -> (w162:u32)
                    n257 = local read "PerformedScans"() -> (w153:dbl)
                    n258 = local read "NrOfScans"() -> (w154:i16)
                    n259 = Subtract(x=w163, y=w162) -> (x-y=w160:u32)
                    n260 = Equal?(x=w153, y=w154) -> (x = y?=w152:bool)
                    n261 = Divide(x=w160, y=u32 1000) -> (x/y=→"TotalTime":dbl)
                    n262 = Divide(x=w160, y=w153) -> (x/y=w157:dbl)
                    "AvgTimePerScan" <- w157
                    n263 = Less Or Equal?(x=w153, y=1.0 ("x")) -> (x <= y?=w159:bool)
                    n264 = case shown="True" w152 {
                      frame #0 {
                      }
                      frame #1 {
                        n265 = property on="StartMeasurement" class="Bool"("Disabled"=u8 0) -> ()  [unwired: 2 in, 2 out]
                      }
                    }
                    n266 = Select(t=w157, s=w159, f=w151) -> (s? t:f=→"LastScanTime":dbl)
                  }
                }
                n267 = call "Convert to Dynamic Data2"("Array"=w120) -> ("Dynamic Data Type"=w119:dynamicdata)  [unwired: 3 in]
                n268 = call "Convert to Dynamic Data"("Array"=w117) -> ("Dynamic Data Type"=w118:dynamicdata)  [unwired: 3 in]
                n269 = call "Build XY Graph"("Y Input"=w119, "X Input"=w118) -> ("XY Graph"=→"XY Graph":cluster{"Y":dbl[], "Y":dbl[]}[])  [unwired: 8 in, 1 out]
              }
            }
          }
        }
        frame #2 {
          n270 = flat-sequence {
            frame #0 {
              n271 = local read "a_hDevice"() -> (w409:i32)
              n272 = property on="StartMeasurement" class="Bool"("Disabled"=u8 0) -> ()  [unwired: 2 in, 2 out]
              n273 = call "AVS_StopMeasure.vi"("a_hDevice"=w409) -> ()  [unwired: 14 in, 1 out]
            }
            frame #1 {
              n274 = local read "a_hDevice"() -> (w411:i32)
              n275 = call "AVS_Deactivate.vi"("a_hHandle"=w411) -> ()  [unwired: 14 in, 1 out]
            }
            frame #2 {
              n276 = call "AVS_Done.vi"() -> ()  [unwired: 19 in, 1 out]
            }
          }
        }
      }
    }
  }
